vi "Configure Multi Eval Meas Limit Inband Emission.vi"(0 "VISA resource name":refnum<visa-resource-name>, 1 "Minimum (-25.0)":dbl=-25.0 format="%^.3e", 2 "RB Power (-55.1)":dbl=-55.1 format="%^.3e", 3 "IQ Image Greater (-25.0)":dbl=-25.0 format="%^.3e", 5 "Instance (1)":T1=1, 7 "Modulation (Pi/2-BPSK)":i32(ring) items=["Pi/2-BPSK", "QPSK", "16-QAM", "64-QAM", "256-QAM"], 9 "Enable (On)":bool=TRUE, 11 "error in (no error)":errorcluster, 12 "EVM (30.0)":dbl=30.0 format="%^.3e", 13 "IQ Image Lesser (-20.0)":dbl=-20.0 format="%^.3e") -> (4 "VISA resource name out":refnum<visa-resource-name>, 15 "error out":errorcluster)   [LabVIEW 2020, in "Rohde&Schwarz CMXP NR FR2 Measurement.lvlib"]
doc: "Defines parameters used for calculation of an upper limit for the inband emission (I/2-BPSK modulation).\n\nAttributes:\nRSCMXPNRFR2M_ATTR_MULTI_EVAL_MEASUREMENT_LIMIT_PHBPSK_INBAND_EMISSION\nRSCMXPNRFR2M_ATTR_MULTI_EVAL_MEASUREMENT_LIMIT_QPSK_INBAND_EMISSION\nRSCMXPNRFR2M_ATTR_MULTI_EVAL_MEASUREMENT_LIMIT_QAM16_INBAND_EMISSION\nRSCMXPNRFR2M_ATTR_MULTI_EVAL_MEASUREMENT_LIMIT_QAM64_INBAND_EMISSION\nRSCMXPNRFR2M_ATTR_MULTI_EVAL_MEASUREMENT_LIMIT_QAM256_INBAND_EMISSION\n\nRemote-control commands:\nCONFigure:NRMMw:MEAS<i>:MEValuation:LIMit:PHBPsk:IBE\nCONFigure:NRMMw:MEAS<i>:MEValuation:LIMit:QPSK:IBE\nCONFigure:NRMMw:MEAS<i>:MEValuation:LIMit:QAM<order>:IBE"
uses:
  <instrlib>/Rohde&Schwarz CMXP NR FR2 Measurement/Rohde&Schwarz CMXP NR FR2 Measurement.lvlib
  <instrlib>/Rohde&Schwarz CMXP NR FR2 Measurement/Private/_Instance.ctl
  <instrlib>/Rohde&Schwarz CMXP NR FR2 Measurement/Private/rsidr_core.llb/rsidr_core.lvlib
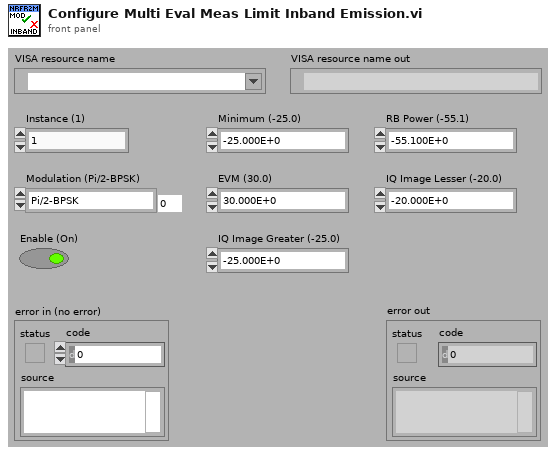
[diagram p1: front panel]
types:
  T1 = typedef "Rohde&Schwarz CMXP NR FR2 Measurement.lvlib/_Instance.ctl" = i32
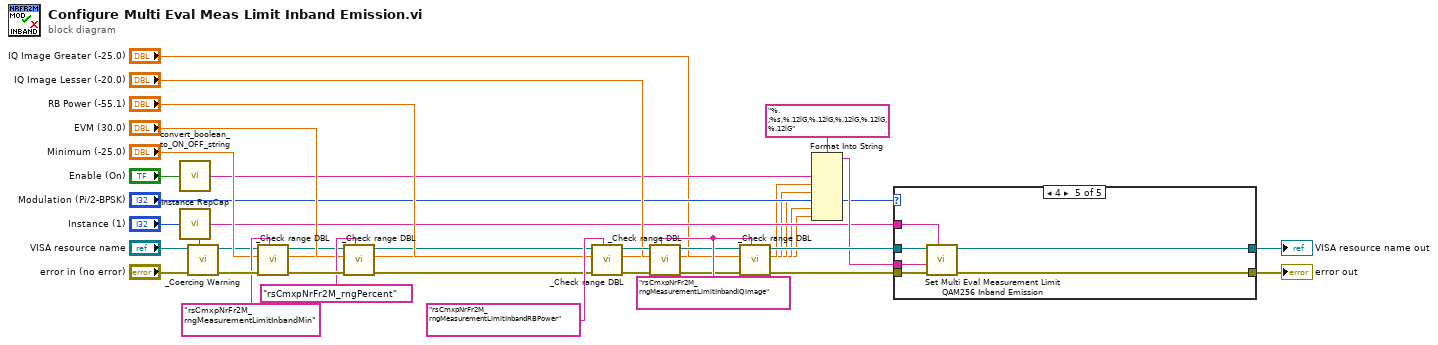
[diagram p0: block diagram]
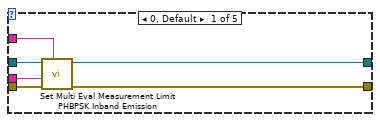
[diagram p2: hidden frame]
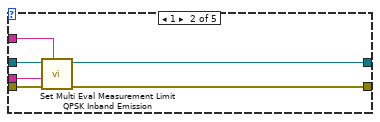
[diagram p3: hidden frame]
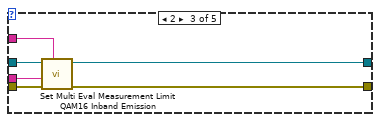
[diagram p4: hidden frame]
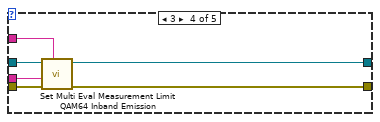
[diagram p5: hidden frame]
diagram:
  w22 = "rsCmxpNrFr2M_rngMeasurementLimitInbandIQImage"
  n1 = call <instrlib>:"convert_boolean_to_ON_OFF_string.vi"("boolean value in"="Enable (On)") -> ("string value out"=w15:string)  [unwired: 4 in]
  n2 = call <instrlib>:"Instance RepCap.vi"("Instance In"="Instance (1)") -> ("In Range?"=w36:bool, "RepCap Identifier Out"=w11:string)  [unwired: 1 in]
  n3 = call <instrlib>:"_Coercing Warning.vi"("In Range?"=w36, "error in (no error)"="error in (no error)", "VISA resource name"="VISA resource name") -> ("error out"=w34:errorcluster, "VISA resource name out"=w27:refnum<visa-resource-name>)  [unwired: 7 in]
  n4 = call <instrlib>:"_Check range DBL.vi"("Range Table Identifier"="rsCmxpNrFr2M_rngMeasurementLimitInbandMin", "error in (no error)"=w34, "DBL Value In"="Minimum (-25.0)", "VISA resource name"=w27) -> ("error out"=w31:errorcluster, "DBL Value Out"=w6:dbl, "VISA resource name out"=w28:refnum<visa-resource-name>)  [unwired: 5 in]
  n5 = call <instrlib>:"_Check range DBL.vi"("Range Table Identifier"="rsCmxpNrFr2M_rngPercent", "error in (no error)"=w31, "DBL Value In"="EVM (30.0)", "VISA resource name"=w28) -> ("error out"=w23:errorcluster, "DBL Value Out"=w5:dbl, "VISA resource name out"=w24:refnum<visa-resource-name>)  [unwired: 5 in]
  n6 = call <instrlib>:"_Check range DBL.vi"("Range Table Identifier"="rsCmxpNrFr2M_rngMeasurementLimitInbandRBPower", "error in (no error)"=w23, "DBL Value In"="RB Power (-55.1)", "VISA resource name"=w24) -> ("error out"=w20:errorcluster, "DBL Value Out"=w4:dbl, "VISA resource name out"=w21:refnum<visa-resource-name>)  [unwired: 5 in]
  n7 = call <instrlib>:"_Check range DBL.vi"("Range Table Identifier"=w22, "error in (no error)"=w20, "DBL Value In"="IQ Image Lesser (-20.0)", "VISA resource name"=w21) -> ("error out"=w17:errorcluster, "DBL Value Out"=w3:dbl, "VISA resource name out"=w18:refnum<visa-resource-name>)  [unwired: 5 in]
  n8 = call <instrlib>:"_Check range DBL.vi"("Range Table Identifier"=w22, "error in (no error)"=w17, "DBL Value In"="IQ Image Greater (-25.0)", "VISA resource name"=w18) -> ("error out"=w13:errorcluster, "DBL Value Out"=w2:dbl, "VISA resource name out"=w14:refnum<visa-resource-name>)  [unwired: 5 in]
  n9 = Format Into String(format string="%.;%s,%.12lG,%.12lG,%.12lG,%.12lG,%.12lG", w15, w6, w5, w4, w3, w2) -> (resulting string=w12:string)  [unwired: 2 in, 1 out]
  n10 = case shown="4" "Modulation (Pi/2-BPSK)" {
    tunnel: w14 -> [w44 w50 w56 w62 w68]
    tunnel: w13 -> [w43 w49 w55 w61 w67]
    tunnel: w12 -> [w39 w45 w51 w57 w63]
    tunnel: w11 -> [w42 w48 w54 w60 w66]
    tunnel: [w41 w47 w53 w59 w65] -> w9
    tunnel: [w40 w46 w52 w58 w64] -> w8
    frame 0, Default {
      n11 = call "Set Multi Eval Measurement Limit PHBPSK Inband Emission"("Repeated Capabilities"=w42, "error in (no error)"=w43, "Multi Eval Measurement Limit PHBPSK Inband Emission ()"=w39, "instrument handle"=w44) -> ("error out"=w41:errorcluster, "instrument handle out"=w40:refnum<visa-resource-name>)  [unwired: 6 in]
    }
    frame 1 {
      n12 = call "Set Multi Eval Measurement Limit QPSK Inband Emission"("Repeated Capabilities"=w48, "error in (no error)"=w49, "Multi Eval Measurement Limit QPSK Inband Emission ()"=w45, "instrument handle"=w50) -> ("error out"=w47:errorcluster, "instrument handle out"=w46:refnum<visa-resource-name>)  [unwired: 6 in]
    }
    frame 2 {
      n13 = call "Set Multi Eval Measurement Limit QAM16 Inband Emission"("Repeated Capabilities"=w54, "error in (no error)"=w55, "Multi Eval Measurement Limit QAM16 Inband Emission ()"=w51, "instrument handle"=w56) -> ("error out"=w53:errorcluster, "instrument handle out"=w52:refnum<visa-resource-name>)  [unwired: 6 in]
    }
    frame 3 {
      n14 = call "Set Multi Eval Measurement Limit QAM64 Inband Emission"("Repeated Capabilities"=w60, "error in (no error)"=w61, "Multi Eval Measurement Limit QAM64 Inband Emission ()"=w57, "instrument handle"=w62) -> ("error out"=w59:errorcluster, "instrument handle out"=w58:refnum<visa-resource-name>)  [unwired: 6 in]
    }
    frame 4 {
      n15 = call "Set Multi Eval Measurement Limit QAM256 Inband Emission"("Repeated Capabilities"=w66, "error in (no error)"=w67, "Multi Eval Measurement Limit QAM256 Inband Emission ()"=w63, "instrument handle"=w68) -> ("error out"=w65:errorcluster, "instrument handle out"=w64:refnum<visa-resource-name>)  [unwired: 6 in]
    }
  }
  "error out" <- w9
  "VISA resource name out" <- w8
